vi "az_to_rad.vi"   [LabVIEW 2015]
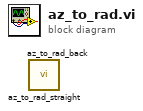
[diagram p0: block diagram]
diagram:
  n1 = call "az_to_rad_straight.vi"() -> ()  [unwired: 2 in, 1 out]
  n2 = call "az_to_rad_back.vi"() -> ()  [unwired: 2 in, 1 out]
